vi "FormatData.vi"(8 "error in (no error)":errorcluster, 9 "Lower Irradiance 2":dbl, 10 "Upper Irradiance":dbl, 11 "Read Buffer":string) -> (0 "error out":errorcluster, 3 "CSV Output":string)   [LabVIEW 2015]
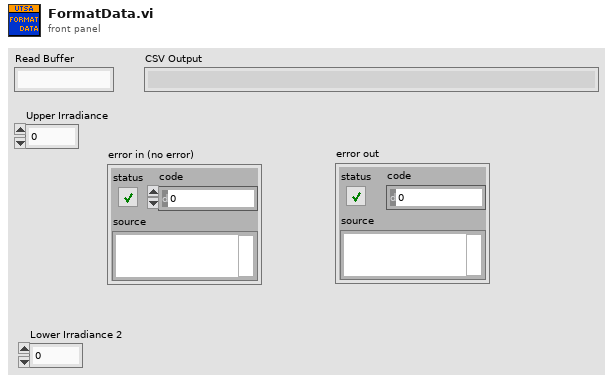
[diagram p1: front panel]
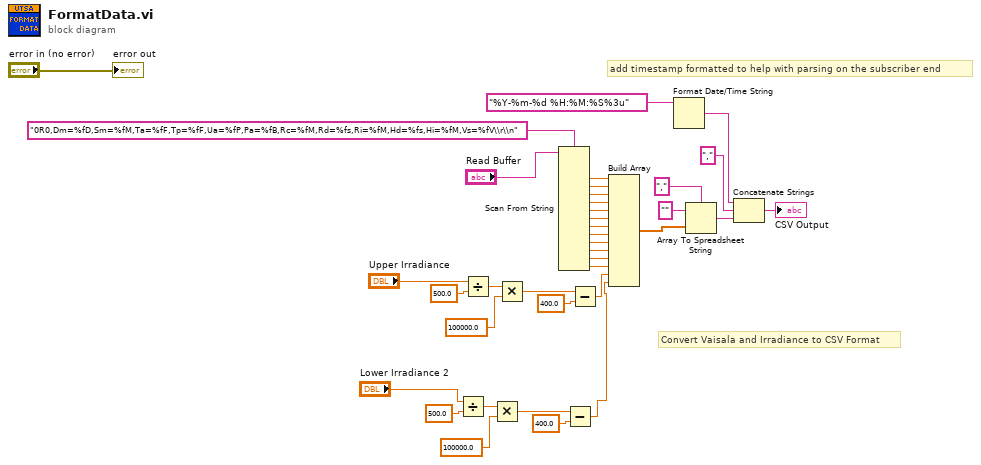
[diagram p0: block diagram]
diagram:
  # "add timestamp formatted to help with parsing on the subscriber end"
  # "Convert Vaisala and Irradiance to CSV Format"
  n1 = Divide(x="Lower Irradiance 2", y=500.0) -> (x/y=w3:dbl)
  n2 = Divide(x="Upper Irradiance", y=500.0) -> (x/y=w18:dbl)
  n3 = Multiply(x=w3, y=100000.0) -> (x*y=w6:dbl)
  n4 = Multiply(x=w18, y=100000.0) -> (x*y=w15:dbl)
  n5 = Scan From String(format string="0R0,Dm=%fD,Sm=%fM,Ta=%fF,Tp=%fF,Ua=%fP,Pa=%fB,Rc=%fM,Rd=%fs,Ri=%fM,Hd=%fs,Hi=%fM,Vs=%fV\\r\\n", input string="Read Buffer") -> (output 1=w33:dbl, output 2=w20:dbl, output 3=w21:dbl, output 4=w22:dbl, output 5=w24:dbl, output 6=w23:dbl, output 7=w25:dbl, output 8=w26:dbl, output 9=w27:dbl, output 10=w19:dbl, output 11=w28:dbl, output 12=w29:dbl)  [unwired: 14 in, 3 out]
  n6 = Subtract(x=w6, y=400.0) -> (x-y=w1:dbl)
  n7 = Subtract(x=w15, y=400.0) -> (x-y=w32:dbl)
  n8 = Build Array(w33, w20, w21, w22, w24, w23, w25, w26, w27, w19, w28, w29, w32, w1) -> (w34:dbl[])
  n9 = Format Date/Time String(time format string (%c)="%Y-%m-%d %H:%M:%S%3u") -> (date/time string=w12:string)  [unwired: 2 in]
  n10 = Array To Spreadsheet String(delimiter (Tab)=",", array=w34, 3:"" ("format string")) -> (spreadsheet string=w10:string)
  n11 = Concatenate Strings(w12, ",", w10) -> (→"CSV Output":string)
  "error out" <- "error in (no error)"
